vi "Init.vi"(8 "error in (no error)":errorcluster, 10 "Name":string, 11 "Process In":refnum<class "Debugger.lvclass">) -> (0 "error out":errorcluster, 3 "Process Out":refnum<class "Debugger.lvclass">)   [LabVIEW 2020, in "Debugger.lvclass"]
doc: "Initializes the process and creates necessary references. Anything initialized here is released in the Clear.vi method."
uses:
  Debugger.lvclass
  State Analyzer/Debug State Analyzer.lvclass
  Debug Latest Message/Debug Latest Message.lvclass
  Debug Log/Debug Log.lvclass
  Debugger.lvclass/Debugger.ctl
  Process/Debug Process.lvclass
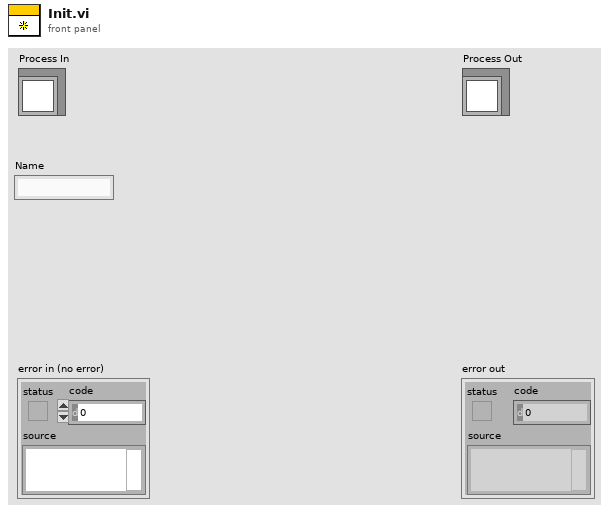
[diagram p1: front panel]
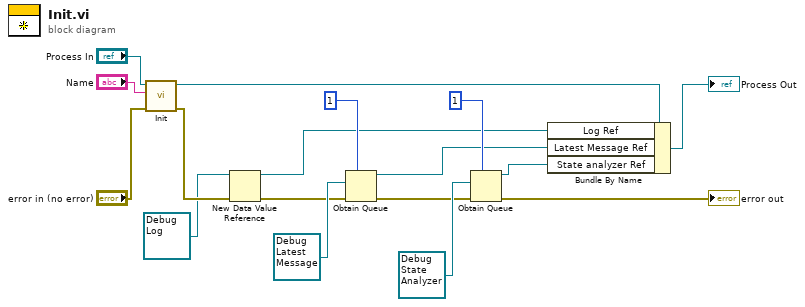
[diagram p0: block diagram]
diagram:
  n1 = call-parent "Init.vi"("error in (no error)"="error in (no error)", "Name"="Name", "Process In"="Process In") -> ("error out"=w17:errorcluster, "Process Out"=w16:refnum<class "Debugger.lvclass">)  [unwired: 7 in]
  n2 = New Data Value Reference(data value=refnum<class "Debug Log.lvclass"> refnum ("Log"), error in=w17) -> (data value reference=w1:refnum<data-value>, error out=w6:errorcluster)
  n3 = Obtain Queue(max queue size (-1, unlimited)=1, element data type=refnum<class "Debug Latest Message.lvclass"> refnum ("Latest Message"), error in (no error)=w6) -> (queue out=w3:refnum<queue>, error out=w5:errorcluster)  [unwired: 2 in, 1 out]
  n4 = Obtain Queue(max queue size (-1, unlimited)=1, element data type=refnum<class "Debug State Analyzer.lvclass"> refnum ("Latest Message"), error in (no error)=w5) -> (queue out=w2:refnum<queue>, error out=→"error out":errorcluster)  [unwired: 2 in, 1 out]
  n5 = Bundle By Name(cluster=w16, "Log Ref"=w1, "Latest Message Ref"=w3, "State analyzer Ref"=w2) -> (→"Process Out":refnum<class "Debugger.lvclass">)
